vi "HTTP_request_buffer.vi"(4 "error in (no error)":errorcluster, 6 "JSON payload":string, 7 "Endpoint":string(combo)="create_folder/") -> (0 "error out":errorcluster, 2 "body":string, 3 "headers":string)   [LabVIEW 2011, in "Rinocloud Library.lvlib"]
uses:
  Rinocloud Library.lvlib
  <vilib>/httpClient/LabVIEWHTTPClient.lvlib
  Rinocloud_global_variable.vi
  <vilib>/httpClient/POSTBuffer.vi
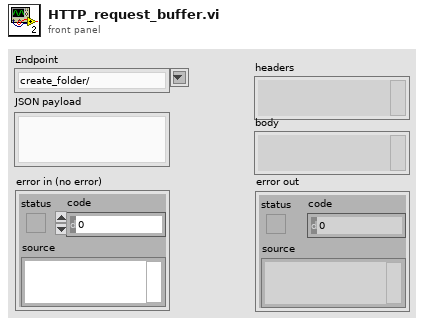
[diagram p1: front panel]
types:
  T1 = typedef "LabVIEWHTTPClient.lvlib/ClientHandle.ctl" = refnum<k1>
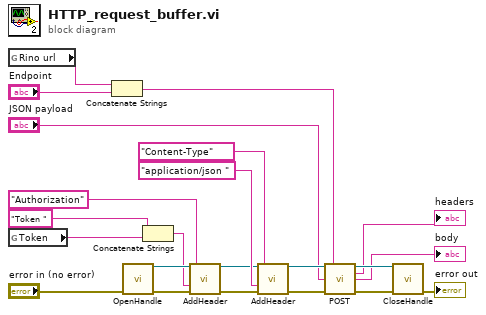
[diagram p0: block diagram]
diagram:
  n1 = global read "Rinocloud_global_variable.vi" "Rino url"() -> (w20:string)
  n2 = global read "Rinocloud_global_variable.vi" "Token"() -> (w14:string)
  n3 = Concatenate Strings(w20, "Endpoint") -> (w22:string)
  n4 = call <vilib>:"OpenHandle.vi"("error in (no error)"="error in (no error)") -> ("client handle out"=w18:T1, "error out"=w15:errorcluster)  [unwired: 13 in]
  n5 = Concatenate Strings("Token " ("value"), w14) -> (w16:string)
  n6 = call <vilib>:"AddHeader.vi"("client handle"=w18, "header"="Authorization" ("url"), "value"=w16, "error in (no error)"=w15) -> ("client handle out"=w7:T1, "error out"=w5:errorcluster)  [unwired: 10 in]
  n7 = call <vilib>:"AddHeader.vi"("client handle"=w7, "header"="Content-Type", "value"="application/json ", "error in (no error)"=w5) -> ("client handle out"=w6:T1, "error out"=w4:errorcluster)  [unwired: 10 in]
  n8 = call-poly <vilib>:"POST.vi"("client handle"=w6, "url"=w22, "buffer"="JSON payload", "error in (no error)"=w4) -> ("client handle out"=w13:T1, "headers"=→"headers":string, "body"=→"body":string, "error out"=w12:errorcluster)  [unwired: 8 in]
  n9 = call <vilib>:"CloseHandle.vi"("client handle"=w13, "error in (no error)"=w12) -> ("error out"=→"error out":errorcluster)  [unwired: 13 in]
